vi "PMX_ClearPeakValues.vi"(0 "Device":refnum<k24>, 1 "Signal":refnum<k24>, 2 "ClearMin":bool=TRUE, 3 "ClearMax":bool=TRUE, 4 "ClearPeakToPeak":bool=TRUE, 5 "Error in":errorcluster) -> (14 "Device":refnum<k24>, 19 "Error out":errorcluster)   [LabVIEW 2016]
doc: "Clears the peak values (min, max, peak to peak) of the given signal.\n\n\nSignal: Signal that holds the peak values\nClearMin: Set to true, if you want to clear the minimum value (default value is true)\nClearMax: Set to true, if you want to clear the maximum value (default value is true)\nClearPeakToPeak: Set to true, if you want to clear the peak to peak value (default value is true)"
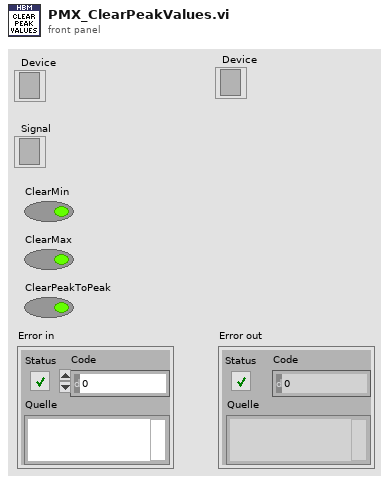
[diagram p1: front panel]
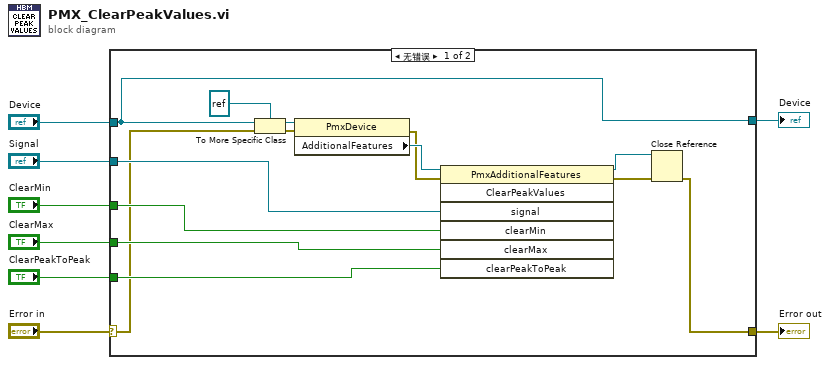
[diagram p0: block diagram]
diagram:
  n1 = case shown="无错误" "Error in" {
    selector: "Error in" -> [w13 w24]
    tunnel: [w9 w24] -> w6
    tunnel: "Device" -> [w18 w23]
    tunnel: [w18 w23] -> w7
    tunnel: "Signal" -> [w17 _]
    tunnel: "ClearPeakToPeak" -> [w16 _]
    tunnel: "ClearMax" -> [w15 _]
    tunnel: "ClearMin" -> [w14 _]
    frame No Error {
      n2 = To More Specific Class(target class=refnum<k24> refnum ("Zielklasse"), reference=w18, error in=w13) -> (specific class reference=w22:refnum<k24>, error out=w19:errorcluster)
      n3 = property on="Eigenschaftsknoten" class="PmxDevice"(reference=w22, error in=w19) -> (error out=w20:errorcluster, "AdditionalFeatures"=w21:refnum<k24>)  [unwired: 1 out]
      n4 = invoke on="Methodenknoten" class="PmxAdditionalFeatures" method="ClearPeakValues"(reference=w21, error in=w20, "signal"=w17, "clearMin"=w14, "clearMax"=w15, "clearPeakToPeak"=w16) -> (reference out=w10:refnum<k24>, error out=w11:errorcluster)  [unwired: 1 in, 5 out]
      n5 = Close Reference(reference=w10, error in (no error)=w11) -> (error out=w9:errorcluster)
    }
    frame Error {
    }
  }
  "Device" <- w7
  "Error out" <- w6
